vi "cw_1_8.vi"() -> ()   [LabVIEW 2022 SP3]
panel:
  out "Out":string
  in  "In":string="test"
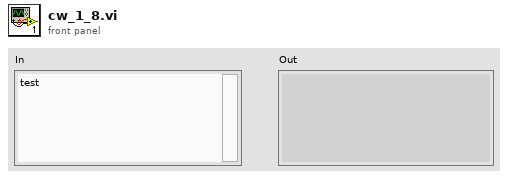
[diagram p1: front panel]
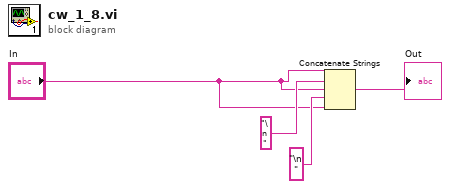
[diagram p0: block diagram]
diagram:
  n1 = Concatenate Strings("In", "\n " ("string"), "In", "\n  " ("string"), "In") -> (→"Out":string)
